vi "Send Set Position.vi"(7 "Priority":T3=enum."Normal" caption="Message Priority (Normal)", 8 "error in (no error)":errorcluster, 9 "Datum":T1, 10 "Target Coordinates":T2, 11 "Message Enqueuer in":refnum<class "Message Enqueuer.lvclass">) -> (0 "error out":errorcluster, 3 "Message Enqueuer out":refnum<class "Message Enqueuer.lvclass">)   [LabVIEW 2014, in "Flex UI (Parent Actor).lvlib" / "Set Position Msg.lvclass"]
doc: "Sends the <b>Set Position Msg.lvclass</b> message.\n\nThis message will call <b>Set Position.vi</b> on the <b>Flex UI (Parent Actor).lvlib:Flex UI (Actor).lvclass</b> actor.\n\n<b>Set Position.vi Description</b>\nWrapper around the set position Flex UI class method."
uses:
  Set Position Msg.lvclass
  <vilib>/ActorFramework/Message Enqueuer/Message Enqueuer.lvclass
  <vilib>/ActorFramework/Message Enqueuer/Message Priority.ctl
  <vilib>/Utility/miscctls.llb/LVPositionTypeDef.ctl
  <vilib>/East West Architects/Flex UI/Flex UI (Parent)/Enum - Datum.ctl
  Set Position Msg.lvclass/Set Position Msg.ctl
  <vilib>/ActorFramework/Message Enqueuer/Message Enqueuer.lvclass/Message Enqueuer.ctl
  <vilib>/ActorFramework/Message Priority Queue/Priority Enqueue.vi
  <vilib>/East West Architects/Flex UI/Flex UI (Parent)/Flex UI.lvclass
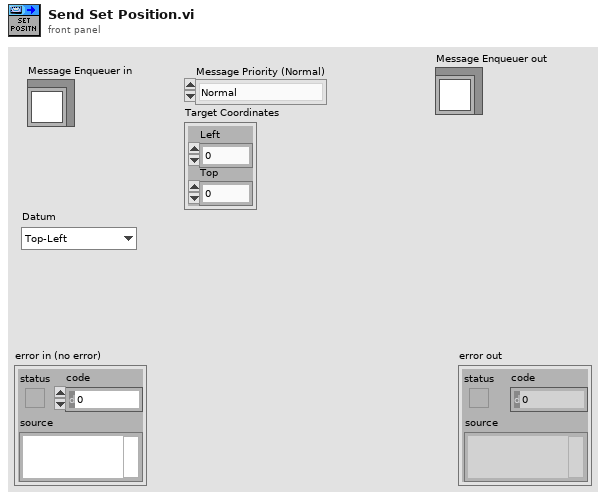
[diagram p1: front panel]
types:
  T1 = typedef "Flex UI.lvclass/Enum - Datum.ctl" = enum16{"Top-Left", "Top-Right", "Bottom-Left", "Bottom-Right", "Center"}
  T2 = typedef "LVPositionTypeDef.ctl" = cluster{"Left":i32, "Top":i32}
  T3 = typedef "Actor Framework.lvlib/Message Enqueuer.lvclass/Message Priority.ctl" = enum16{"Low", "Normal", "High"}
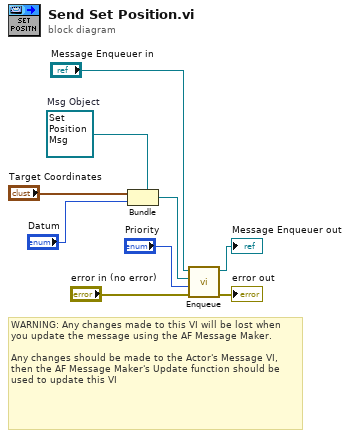
[diagram p0: block diagram]
diagram:
  w8 = refnum<class "Set Position Msg.lvclass"> refnum  # Msg Object
  # "WARNING: Any changes made to this VI will be lost when you update the message using the AF Message Maker.\n\nAny changes should be made to the Actor's Message VI, then the AF Message Maker's Update function should be used to update this VI"
  n1 = Bundle(cluster=w8, "Target Coordinates", "Datum") -> (w3:refnum<class "Set Position Msg.lvclass">)
  n2 = call <vilib>:"Enqueue.vi"("error in (no error)"="error in (no error)", "Message Priority (Normal)"="Priority", "Message"=w3, "Message Enqueuer in"="Message Enqueuer in") -> ("error out"=→"error out":errorcluster, "Message Enqueuer out"=→"Message Enqueuer out":refnum<class "Message Enqueuer.lvclass">)  [unwired: 6 in]
